vi "AnalogDemultiplex_AND_FIXED_samples.vi"(0 "Analog data cluster":T1, 5 "Over? Array":bool[](array[boolean])=[FALSE, FALSE, FALSE, FALSE, FALSE, FALSE, FALSE, FALSE], 7 "Last Sample A1":u8, 9 "Last Sample A2":u8, 11 "Last? Input":bool, 12 "array in":bool[](array[boolean])=[FALSE, FALSE, FALSE, FALSE, FALSE, FALSE, FALSE, FALSE, FALSE, FALSE, FALSE, FALSE, FALSE]) -> (4 "Data A1 out":u64, 6 "Data A2 out":u64, 14 "array out":bool[](array[boolean]), 15 "Last? Output":bool)   [LabVIEW 2014]
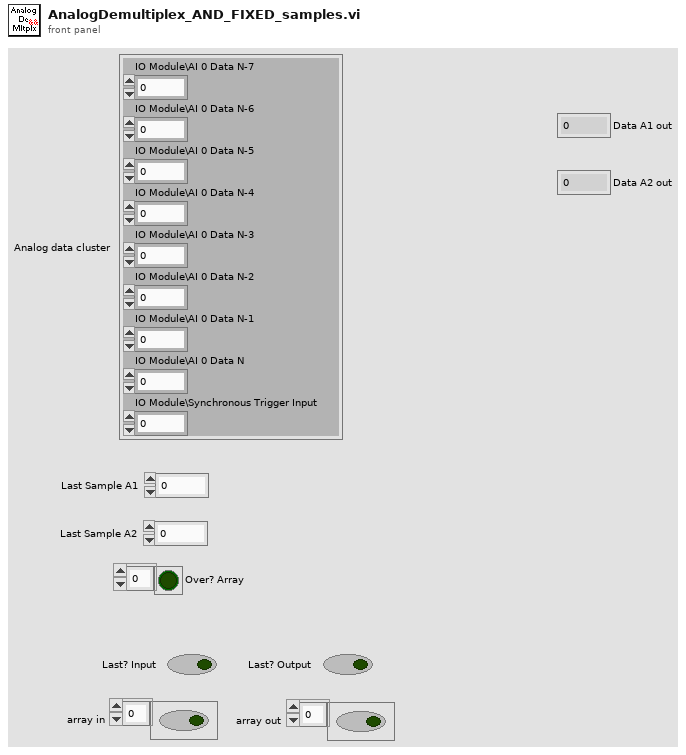
[diagram p1: front panel]
types:
  T1 = cluster{"IO Module\\AI 0 Data N-7":u8, "IO Module\\AI 0 Data N-6":u8, "IO Module\\AI 0 Data N-5":u8, "IO Module\\AI 0 Data N-4":u8, "IO Module\\AI 0 Data N-3":u8, "IO Module\\AI 0 Data N-2":u8, "IO Module\\AI 0 Data N-1":u8, "IO Module\\AI 0 Data N":u8, "IO Module\\Synchronous Trigger Input":u8}
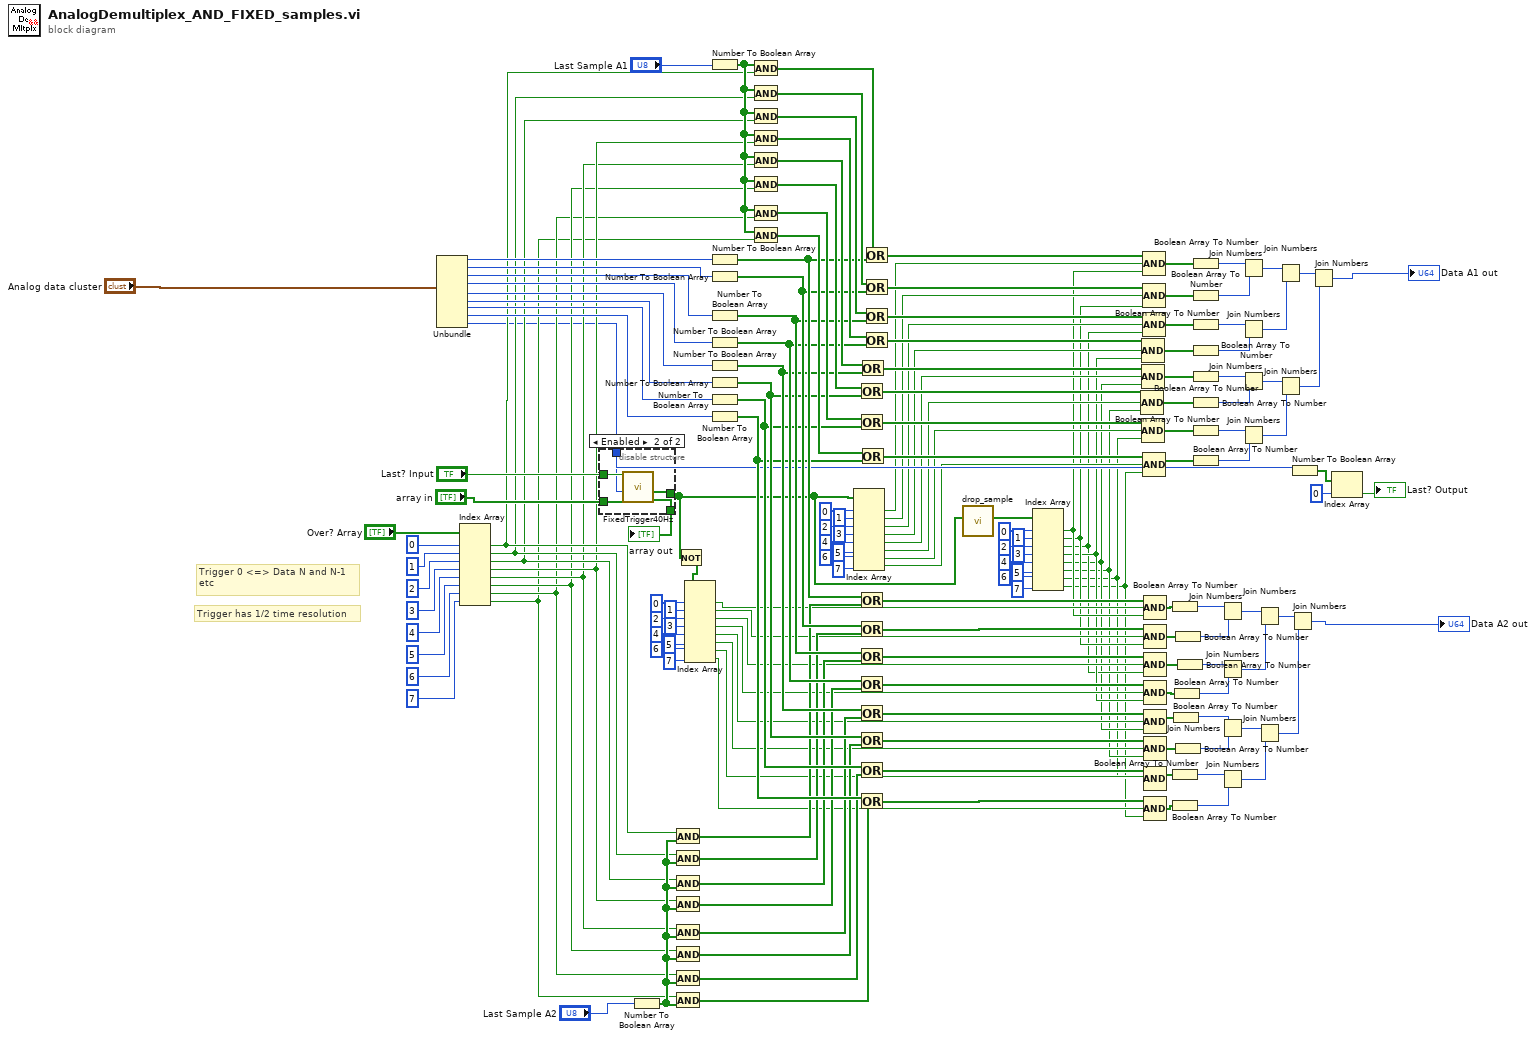
[diagram p0: block diagram]
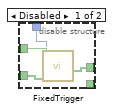
[diagram p2: hidden frame]
diagram:
  # "Trigger 0 <=> Data N and N-1\netc"
  # "Trigger has 1/2 time resolution"
  n1 = Unbundle("Analog data cluster") -> ("IO Module\\AI 0 Data N-7"=w132:u8, "IO Module\\AI 0 Data N-6"=w131:u8, "IO Module\\AI 0 Data N-5"=w130:u8, "IO Module\\AI 0 Data N-4"=w129:u8, "IO Module\\AI 0 Data N-3"=w128:u8, "IO Module\\AI 0 Data N-2"=w127:u8, "IO Module\\AI 0 Data N-1"=w126:u8, "IO Module\\AI 0 Data N"=w125:u8, "IO Module\\Synchronous Trigger Input"=w49:u8)
  n2 = Index Array(array="Over? Array", index #1=0 ("index"), index #2=1 ("index"), index #3=2 ("index"), index #4=3 ("index"), index #5=4 ("index"), index #6=5 ("index"), index #7=6 ("index"), index #8=7 ("index")) -> (element #1=w99:bool, element #2=w98:bool, element #3=w97:bool, element #4=w96:bool, element #5=w95:bool, element #6=w94:bool, element #7=w93:bool, element #8=w92:bool)
  n3 = disable-structure shown="Enabled" {
    disable-tunnel: "Last? Input" -> [w178 w183]
    disable-tunnel: "array in" -> [w177 w181]
    disable-tunnel: [_ w179] -> w169
    disable-tunnel: w49 -> [w176 w182]
    disable-tunnel: [w175 w180] -> w18
    frame Disabled {
      n4 = call "FixedTrigger.vi"("array in"=w177, "IO Module\\Synchronous Trigger Input"=w176, "Last? Input"=w178) -> ("trigger out"=w175:bool[])  [unwired: 7 in, 1 out]
    }
    frame Enabled {
      n5 = call "FixedTrigger40Hz.vi"("array in"=w181, "IO Module\\Synchronous Trigger Input"=w182, "Last? Input"=w183) -> ("array out"=w179:bool[], "trigger out"=w180:bool[])  [unwired: 7 in]
    }
  }
  "array out" <- w169
  n6 = Number To Boolean Array(number="Last Sample A2") -> (Boolean array=w100:bool[])
  n7 = And(x=w99, y=w100) -> (x .and. y?=w59:bool[])
  n8 = And(x=w98, y=w100) -> (x .and. y?=w58:bool[])
  n9 = And(x=w97, y=w100) -> (x .and. y?=w57:bool[])
  n10 = And(x=w96, y=w100) -> (x .and. y?=w56:bool[])
  n11 = And(x=w95, y=w100) -> (x .and. y?=w52:bool[])
  n12 = And(x=w94, y=w100) -> (x .and. y?=w53:bool[])
  n13 = And(x=w93, y=w100) -> (x .and. y?=w54:bool[])
  n14 = And(x=w92, y=w100) -> (x .and. y?=w55:bool[])
  n15 = Not(x=w18) -> (.not. x?=w44:bool[])
  n16 = Index Array(array=w44, index #1=0 ("index"), index #2=1 ("index"), index #3=2 ("index"), index #4=3 ("index"), index #5=4 ("index"), index #6=5 ("index"), index #7=6 ("index"), index #8=7 ("index")) -> (element #1=w43:bool, element #2=w42:bool, element #3=w41:bool, element #4=w40:bool, element #5=w39:bool, element #6=w38:bool, element #7=w37:bool, element #8=w36:bool)
  n17 = Number To Boolean Array(number="Last Sample A1") -> (Boolean array=w101:bool[])
  n18 = Number To Boolean Array(number=w132) -> (Boolean array=w75:bool[])
  n19 = Number To Boolean Array(number=w131) -> (Boolean array=w74:bool[])
  n20 = Number To Boolean Array(number=w130) -> (Boolean array=w73:bool[])
  n21 = Number To Boolean Array(number=w129) -> (Boolean array=w72:bool[])
  n22 = Number To Boolean Array(number=w128) -> (Boolean array=w71:bool[])
  n23 = Number To Boolean Array(number=w127) -> (Boolean array=w70:bool[])
  n24 = Number To Boolean Array(number=w126) -> (Boolean array=w69:bool[])
  n25 = Number To Boolean Array(number=w125) -> (Boolean array=w68:bool[])
  n26 = And(x=w101, y=w99) -> (x .and. y?=w76:bool[])
  n27 = And(x=w101, y=w98) -> (x .and. y?=w77:bool[])
  n28 = And(x=w101, y=w97) -> (x .and. y?=w78:bool[])
  n29 = And(x=w101, y=w96) -> (x .and. y?=w79:bool[])
  n30 = And(x=w101, y=w95) -> (x .and. y?=w80:bool[])
  n31 = And(x=w101, y=w94) -> (x .and. y?=w81:bool[])
  n32 = And(x=w101, y=w93) -> (x .and. y?=w82:bool[])
  n33 = And(x=w101, y=w92) -> (x .and. y?=w83:bool[])
  n34 = Index Array(array=w18, index #1=0 ("index"), index #2=1 ("index"), index #3=2 ("index"), index #4=3 ("index"), index #5=4 ("index"), index #6=5 ("index"), index #7=6 ("index"), index #8=7 ("index")) -> (element #1=w26:bool, element #2=w25:bool, element #3=w24:bool, element #4=w23:bool, element #5=w22:bool, element #6=w21:bool, element #7=w20:bool, element #8=w19:bool)
  n35 = Or(x=w81, y=w70) -> (x .or. y?=w89:bool[])
  n36 = Or(x=w82, y=w69) -> (x .or. y?=w90:bool[])
  n37 = Or(x=w75, y=w59) -> (x .or. y?=w67:bool[])
  n38 = Or(x=w74, y=w58) -> (x .or. y?=w66:bool[])
  n39 = Or(x=w73, y=w57) -> (x .or. y?=w65:bool[])
  n40 = Or(x=w72, y=w56) -> (x .or. y?=w64:bool[])
  n41 = Or(x=w71, y=w52) -> (x .or. y?=w63:bool[])
  n42 = Or(x=w70, y=w53) -> (x .or. y?=w62:bool[])
  n43 = Or(x=w69, y=w54) -> (x .or. y?=w61:bool[])
  n44 = Or(x=w68, y=w55) -> (x .or. y?=w60:bool[])
  n45 = Or(x=w80, y=w71) -> (x .or. y?=w88:bool[])
  n46 = Or(x=w83, y=w68) -> (x .or. y?=w91:bool[])
  n47 = Or(x=w76, y=w75) -> (x .or. y?=w84:bool[])
  n48 = Or(x=w77, y=w74) -> (x .or. y?=w85:bool[])
  n49 = Or(x=w78, y=w73) -> (x .or. y?=w86:bool[])
  n50 = Or(x=w79, y=w72) -> (x .or. y?=w87:bool[])
  n51 = call "drop_sample.vi"("trigger in"=w18) -> ("drop sample"=w9:bool[])  [unwired: 10 in]
  n52 = Index Array(array=w9, index #1=0 ("index"), index #2=1 ("index"), index #3=2 ("index"), index #4=3 ("index"), index #5=4 ("index"), index #6=5 ("index"), index #7=6 ("index"), index #8=7 ("index")) -> (element #1=w8:bool, element #2=w7:bool, element #3=w5:bool, element #4=w6:bool, element #5=w4:bool, element #6=w3:bool, element #7=w2:bool, element #8=w1:bool)
  n53 = Compound Arithmetic op=AND(w89, w21, w3) -> (w114:bool[])
  n54 = Compound Arithmetic op=AND(w87, w23, w6) -> (w113:bool[])
  n55 = Compound Arithmetic op=AND(w88, w22, w4) -> (w142:bool[])
  n56 = Compound Arithmetic op=AND(w90, w20, w2) -> (w143:bool[])
  n57 = Compound Arithmetic op=AND(w84, w26, w8) -> (w139:bool[])
  n58 = Compound Arithmetic op=AND(w85, w25, w7) -> (w120:bool[])
  n59 = Compound Arithmetic op=AND(w86, w24, w5) -> (w141:bool[])
  n60 = Compound Arithmetic op=AND(w91, w19, w1) -> (w115:bool[])
  n61 = Compound Arithmetic op=AND(w67, w43, w8) -> (w165:bool[])
  n62 = Compound Arithmetic op=AND(w66, w42, w7) -> (w116:bool[])
  n63 = Compound Arithmetic op=AND(w65, w41, w5) -> (w166:bool[])
  n64 = Compound Arithmetic op=AND(w64, w40, w6) -> (w117:bool[])
  n65 = Compound Arithmetic op=AND(w63, w39, w4) -> (w167:bool[])
  n66 = Compound Arithmetic op=AND(w62, w38, w3) -> (w118:bool[])
  n67 = Compound Arithmetic op=AND(w61, w37, w2) -> (w168:bool[])
  n68 = Compound Arithmetic op=AND(w60, w36, w1) -> (w119:bool[])
  n69 = Boolean Array To Number(Boolean array=w165) -> (number=w157:u8)
  n70 = Boolean Array To Number(Boolean array=w168) -> (number=w163:u8)
  n71 = Boolean Array To Number(Boolean array=w119) -> (number=w164:u8)
  n72 = Boolean Array To Number(Boolean array=w167) -> (number=w161:u8)
  n73 = Boolean Array To Number(Boolean array=w117) -> (number=w160:u8)
  n74 = Boolean Array To Number(Boolean array=w116) -> (number=w158:u8)
  n75 = Boolean Array To Number(Boolean array=w118) -> (number=w162:u8)
  n76 = Boolean Array To Number(Boolean array=w166) -> (number=w159:u8)
  n77 = Boolean Array To Number(Boolean array=w139) -> (number=w140:u8)
  n78 = Boolean Array To Number(Boolean array=w120) -> (number=w144:u8)
  n79 = Boolean Array To Number(Boolean array=w141) -> (number=w145:u8)
  n80 = Boolean Array To Number(Boolean array=w113) -> (number=w146:u8)
  n81 = Boolean Array To Number(Boolean array=w142) -> (number=w147:u8)
  n82 = Boolean Array To Number(Boolean array=w114) -> (number=w148:u8)
  n83 = Boolean Array To Number(Boolean array=w143) -> (number=w149:u8)
  n84 = Boolean Array To Number(Boolean array=w115) -> (number=w150:u8)
  n85 = Join Numbers(hi=w157, lo=w158) -> ((hi.lo)=w151:u16)
  n86 = Join Numbers(hi=w159, lo=w160) -> ((hi.lo)=w152:u16)
  n87 = Join Numbers(hi=w161, lo=w162) -> ((hi.lo)=w153:u16)
  n88 = Join Numbers(hi=w163, lo=w164) -> ((hi.lo)=w154:u16)
  n89 = Join Numbers(hi=w140, lo=w144) -> ((hi.lo)=w133:u16)
  n90 = Join Numbers(hi=w145, lo=w146) -> ((hi.lo)=w134:u16)
  n91 = Join Numbers(hi=w147, lo=w148) -> ((hi.lo)=w135:u16)
  n92 = Join Numbers(hi=w149, lo=w150) -> ((hi.lo)=w136:u16)
  n93 = Join Numbers(hi=w151, lo=w152) -> ((hi.lo)=w156:u32)
  n94 = Join Numbers(hi=w153, lo=w154) -> ((hi.lo)=w155:u32)
  n95 = Join Numbers(hi=w133, lo=w134) -> ((hi.lo)=w138:u32)
  n96 = Join Numbers(hi=w135, lo=w136) -> ((hi.lo)=w137:u32)
  n97 = Join Numbers(hi=w156, lo=w155) -> ((hi.lo)=→"Data A2 out":u64)
  n98 = Number To Boolean Array(number=w49) -> (Boolean array=w50:bool[])
  n99 = Join Numbers(hi=w138, lo=w137) -> ((hi.lo)=→"Data A1 out":u64)
  n100 = Index Array(array=w50, index=0) -> (element=→"Last? Output":bool)
